vi "Set Cursor Position.vi"(8 "error in (no error)":errorcluster, 10 "Cursor.Cursor Position":T1, 11 "Graph Ref In":refnum<vi>) -> (0 "error out":errorcluster, 3 "Graph Ref Out":refnum<vi>)   [LabVIEW 2019, in "Graph Tools.lvlib"]
doc: "Set Cursor Position."
uses:
  Graph Tools.lvlib
  <vilib>/Utility/miscctls.llb/LVPointDoubleTypeDef.ctl
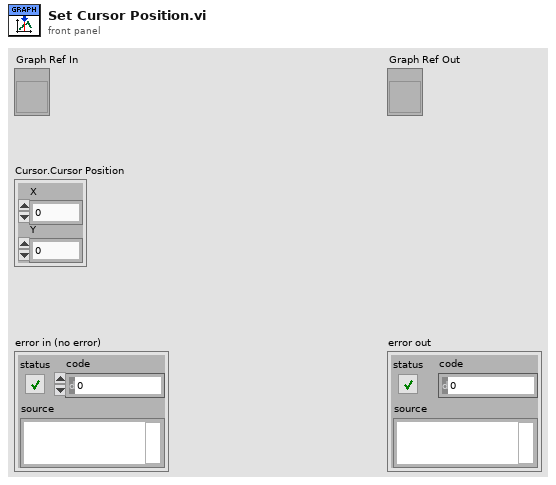
[diagram p1: front panel]
types:
  T1 = typedef "LVPointDoubleTypeDef.ctl" = cluster{"X":dbl, "Y":dbl}
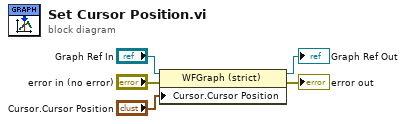
[diagram p0: block diagram]
diagram:
  n1 = property on="Property Node" class="WFGraph (strict)"(reference="Graph Ref In", error in="error in (no error)", "Cursor.Cursor Position"="Cursor.Cursor Position") -> (reference out=→"Graph Ref Out":refnum<vi>, error out=→"error out":errorcluster)
